vi "Click Cycle_Get Current Row State.vi"(8 "error in":errorcluster, 10 "Active Item:Tag":string, 11 "All Tree Refs":refnum<vi>[](array[refnum])) -> (0 "error out":errorcluster, 2 "Row RW State":T1, 3 "All Tree Refs Out":refnum<vi>[](array[refnum]))   [LabVIEW 2023]
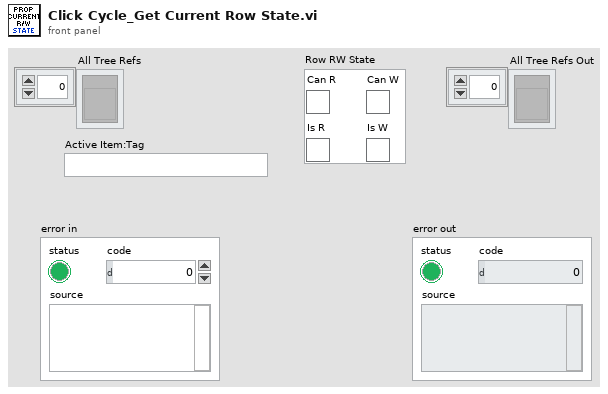
[diagram p1: front panel]
types:
  T1 = cluster{"Can R":bool, "Can W":bool, "Is R":bool, "Is W":bool}
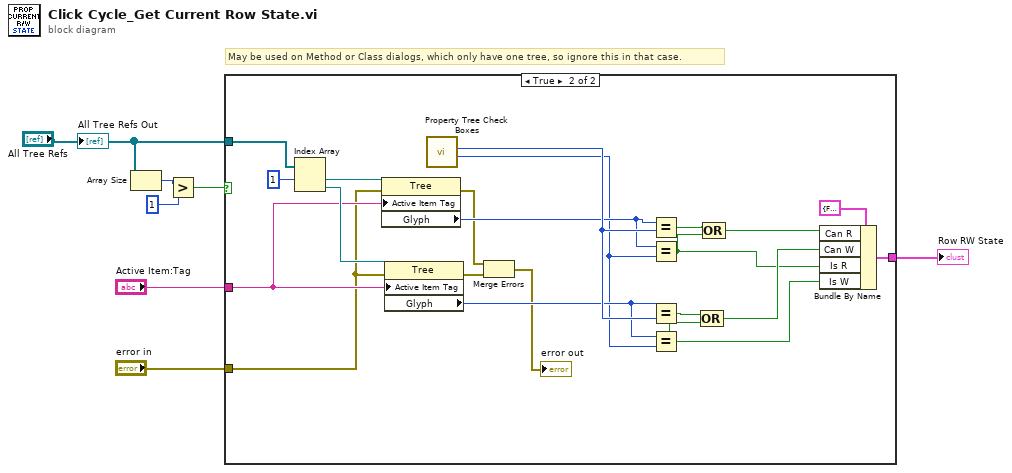
[diagram p0: block diagram]
diagram:
  # "May be used on Method or Class dialogs, which only have one tree, so ignore this in that case."
  n1 = Array Size(array="All Tree Refs") -> (size(s)=w3:i32)
  n2 = Greater?(x=w3, y=1) -> (0:w1:bool)
  n3 = case shown="True" w1 {
    tunnel: "Active Item:Tag" -> [_ w25]
    tunnel: [_ w18] -> w6
    tunnel: "error in" -> [_ w12]
    tunnel: "All Tree Refs" -> [_ w8]
    frame False {
    }
    frame True {
      n4 = Index Array(array=w8, index #1=1 ("index")) -> (element #1=w27:refnum<vi>, element #2=w26:refnum<vi>)  [unwired: 1 in]
      n5 = property class="Tree"(reference=w27, error in=w12, "Active Item Tag"=w25) -> (error out=w10:errorcluster, "Glyph"=w22:i32)  [unwired: 1 out]
      n6 = property class="Tree"(reference=w26, error in=w12, "Active Item Tag"=w25) -> (error out=w11:errorcluster, "Glyph"=w23:i32)  [unwired: 1 out]
      n7 = call "Property Tree Check Boxes.vi"() -> ("Checked"=w21:i32, "Unchecked"=w24:i32)  [unwired: 9 in, 1 out]
      n8 = Merge Errors(w10, w11) -> (→"error out":errorcluster)
      n9 = Equal?(x=w22, y=w24) -> (x = y?=w20:bool)
      n10 = Equal?(x=w22, y=w21) -> (x = y?=w14:bool)
      n11 = Equal?(x=w23, y=w24) -> (x = y?=w19:bool)
      n12 = Equal?(x=w23, y=w21) -> (x = y?=w13:bool)
      n13 = Compound Arithmetic op=OR(w19, w13) -> (w15:bool)
      n14 = Compound Arithmetic op=OR(w20, w14) -> (w16:bool)
      n15 = Bundle By Name(cluster=T1 {"Can R"=FALSE, "Can W"=FALSE, "Is R"=FALSE, "Is W"=FALSE} ("Row RW State"), "Can R"=w16, "Can W"=w15, "Is R"=w14, "Is W"=w13) -> (w18:T1)
    }
  }
  "Row RW State" <- w6
  "All Tree Refs Out" <- "All Tree Refs"
